vi "Boolean To AStar Map.vi"(1 "empty value":dbl, 2 "Wall value":dbl, 3 "Obstacles":bool[][](array[boolean])) -> (0 "a star map":dbl[][](array[numeric]))   [LabVIEW 2015]
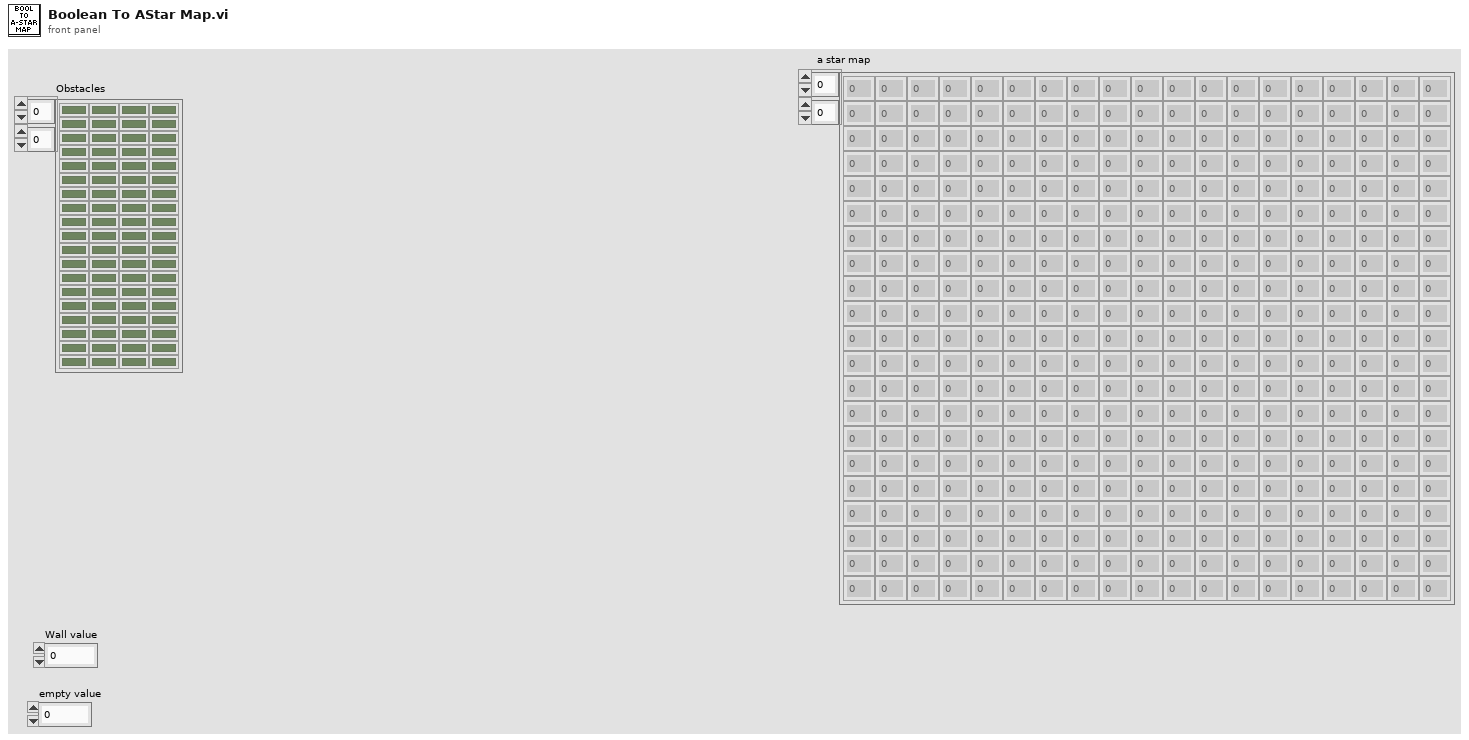
[diagram p1: front panel]
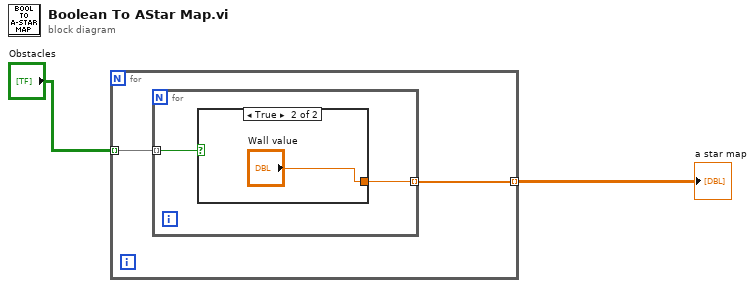
[diagram p0: block diagram]
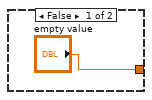
[diagram p2: hidden frame]
diagram:
  n1 = for {
    tunnel: "Obstacles" -> [w4] mode=indexing
    tunnel: [w3] -> w1 mode=indexing
    n2 = for {
      tunnel: w4 -> [w6] mode=indexing
      tunnel: [w5] -> w3 mode=indexing
      n3 = case shown="True" w6 {
        tunnel: ["empty value" "Wall value"] -> w5
        frame False {
        }
        frame True {
        }
      }
    }
  }
  "a star map" <- w1
